vi "user32_mouse_move.vi"(11 "VI输入":refnum<vi>) -> ()   [LabVIEW 2017]
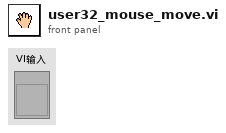
[diagram p1: front panel]
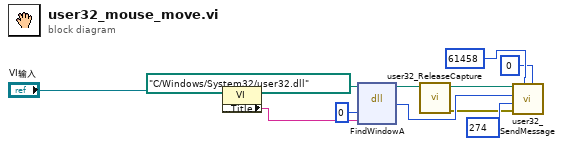
[diagram p0: block diagram]
diagram:
  n1 = property class="VI"(reference="VI输入") -> ("Front Panel.Title"=w4:string)  [unwired: 1 in, 2 out]
  n2 = dll-call lib="PTH2Jabs D迈致项目资料MovellaFttWINDOWSSYSTEM32\nuser32.dll" fn="FindWindowA"(path in=path "C:/Windows/System32/user32.dll" ("路径输入"), "lpszClassName"=0, "lpszWindowName"=w4) -> (path out=w6:path, "hWnd"=w9:u32)  [unwired: 4 in, 1 out]
  n3 = call "user32_ReleaseCapture.vi"("路径输入"=w6) -> ("错误输出"=w1:errorcluster, "路径输出"=w7:path)  [unwired: 8 in, 1 out]
  n4 = call "user32_SendMessage.vi"("IParam"=u32 0, "wParam"=u32 61458 ("IParam"), "错误输入（无错误）"=w1, "Msg"=u32 274 ("IParam"), "hWnd"=w9, "路径输入"=w7) -> ()  [unwired: 4 in, 2 out]
